vi "Arduino to LabVIEW Communication Module JSON.vi"() -> ()   [LabVIEW 2018]
uses:
  TypeDeclarations/GEVE Ventilator Monitoring Data.ctl
  <vilib>/Instr/_visa.llb/VISA Configure Serial Port (Instr).vi
panel:
  out "GEVE Ventilator Monitoring Data":T1
  out "loop time (ms)":u32
  out "Waveform Chart":u32(graph)
  out "read buffer data byte array":u8[](array[numeric]) format="%02x"
  in  "baud rate (9600)":u32=9600
  out "Communication Timeout?":bool
  in  "VISA resource name":refnum<visa-resource-name>="COM7"
  out "return count read":u32
  out "read buffer":string
  in  "Stop":bool
  out "Iterations":i32
  # "DEBUG AREA"
  # "iterations"
  # "poti"
  # "pressure"
  # "alarm"
  # "EOL"
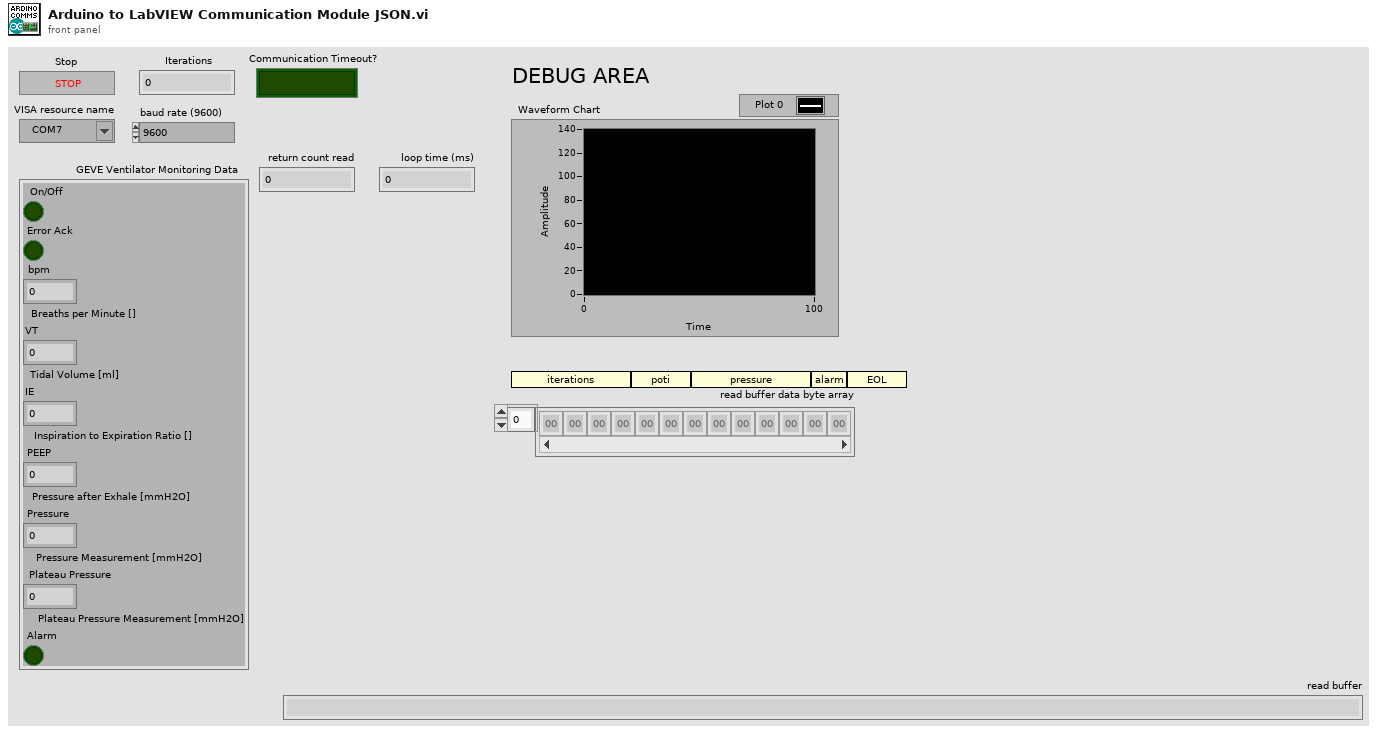
[diagram p1: front panel]
types:
  T1 = typedef "GEVE Ventilator Monitoring Data.ctl" = cluster{"On/Off":bool, "Error Ack":bool, "bpm":dbl, "VT":dbl, "IE":dbl, "PEEP":dbl, "Pressure":dbl, "Plateau Pressure":dbl, "Alarm":bool}
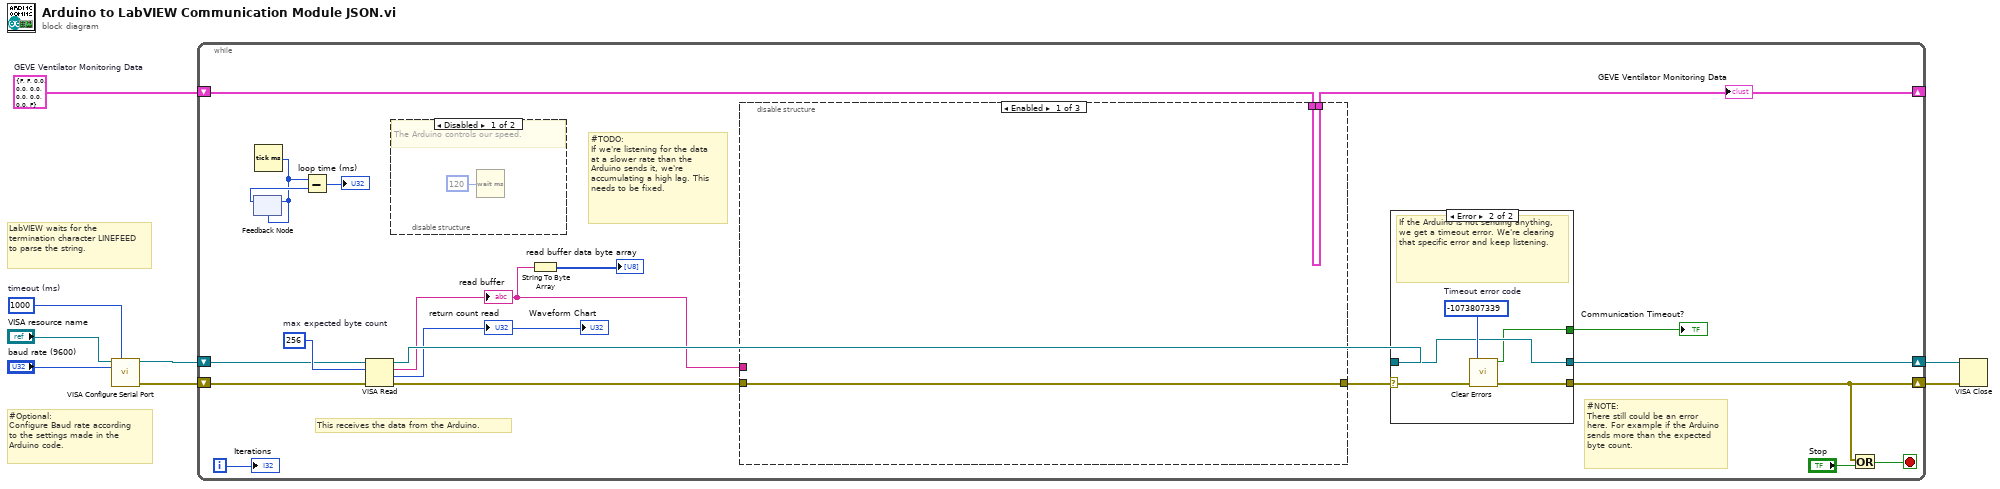
[diagram p0: block diagram]
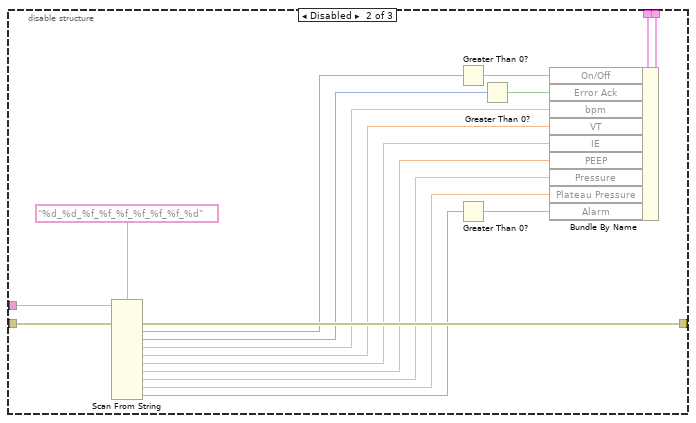
[diagram p2: hidden frame]
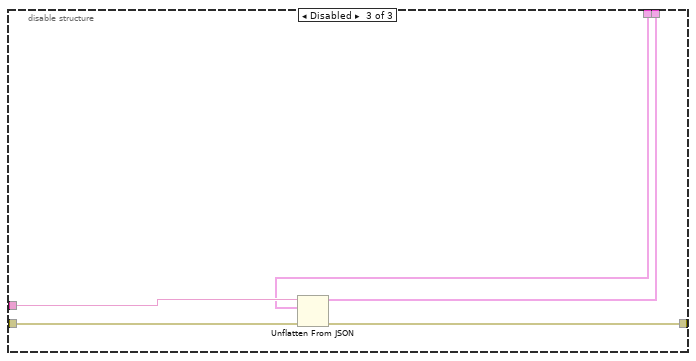
[diagram p3: hidden frame]
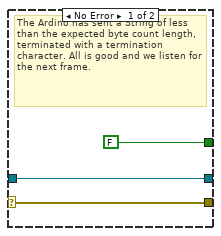
[diagram p5: hidden frame]
diagram:
  w1 = T1 {"On/Off"=FALSE, "Error Ack"=FALSE, "bpm"=0.0, "VT"=0.0, "IE"=0.0, "PEEP"=0.0, "Pressure"=0.0, "Plateau Pressure"=0.0, "Alarm"=FALSE}  # GEVE Ventilator Monitoring Data
  w3 = u32 1000  # timeout (ms)
  # "#Optional:\nConfigure Baud rate according to the settings made in the Arduino code."
  # "LabVIEW waits for the termination character LINEFEED to parse the string."
  n1 = call-poly "VISA Configure Serial Port"("VISA resource name"="VISA resource name", "timeout (10sec)"=w3, "baud rate (9600)"="baud rate (9600)") -> ("VISA resource name out"=w8:refnum<visa-resource-name>, "error out"=w6:errorcluster)  [unwired: 11 in]
  n2 = while {
    shift-right: [w23] -> w7
    shift-left: w8 -> [w12]
    shift-right: [w24] -> w5
    shift-left: w6 -> [w11]
    shift-right: [w9] -> _
    shift-left: w1 -> [w10]
    i -> [w28]
    stop <- w26 stop-if-true
    w25 = u32 256  # max expected byte count
    # "#TODO:\nIf we're listening for the data at a slower rate than the Arduino sends it, we're accumulating a high lag. This needs to be fixed."
    # "This receives the data from the Arduino."
    # "#NOTE:\nThere still could be an error here. For example if the Arduino sends more than the expected byte count."
    n3 = Tick Count (ms)() -> (millisecond timer value=w13:u32)
    n4 = feedback #1(w13) -> (w15:u32)
    n5 = feedback-in #1(w13) -> ()
    n6 = Subtract(x=w13, y=w15) -> (x-y=→"loop time (ms)":u32)
    n7 = VISA Read(VISA resource name=w12, byte count=w25, error in (no error)=w11) -> (VISA resource name out=w22:refnum<visa-resource-name>, read buffer=w17:string, return count=→"return count read" →"Waveform Chart":u32, error out=w16:errorcluster)
    "read buffer" <- w17
    n8 = disable-structure shown="Disabled" {
      frame Disabled {
        # "The Arduino controls our speed."
        n9 = Wait (ms)(milliseconds to wait=u32 120) -> ()  [unwired: 1 out]
      }
      frame Enabled {
      }
    }
    n10 = String To Byte Array(string=w17) -> (unsigned byte array=→"read buffer data byte array":u8[])
    n11 = disable-structure shown="Enabled" {
      disable-tunnel: [w30 w48 w52] -> w20
      disable-tunnel: w17 -> [_ w47 w51]
      disable-tunnel: w16 -> [w30 w46 w53]
      disable-tunnel: w10 -> [w29 w43 w50]
      disable-tunnel: [w29 w42 w49] -> w9
      frame Enabled {
      }
      frame Disabled {
        n12 = Scan From String(format string="%d_%d_%f_%f_%f_%f_%f_%f_%d", input string=w47, error in=w46) -> (error out=w48:errorcluster, output 1=w40:i32, output 2=w39:i32, output 3=w44:dbl, output 4=w31:dbl, output 5=w32:dbl, output 6=w33:dbl, output 7=w34:dbl, output 8=w35:dbl, output 9=w41:i32)  [unwired: 10 in, 2 out]
        n13 = Greater Than 0?(x=w40) -> (x > 0?=w38:bool)
        n14 = Greater Than 0?(x=w41) -> (x > 0?=w36:bool)
        n15 = Greater Than 0?(x=w39) -> (x > 0?=w37:bool)
        n16 = Bundle By Name(cluster=w43, "On/Off"=w38, "Error Ack"=w37, "bpm"=w44, "VT"=w31, "IE"=w32, "PEEP"=w33, "Pressure"=w34, "Plateau Pressure"=w35, "Alarm"=w36) -> (w42:T1)
      }
      frame Disabled {
        n17 = Unflatten From JSON(JSON string=w51, type and defaults=w50, error in (no error)=w53) -> (value=w49:T1, error out=w52:errorcluster)  [unwired: 4 in]
      }
    }
    "GEVE Ventilator Monitoring Data" <- w9
    n18 = case shown="Error" w20 {
      selector: w20 -> [w57 w62]
      tunnel: [w57 w60] -> w24
      tunnel: [w56 w59] -> w23
      tunnel: w22 -> [w56 w59]
      tunnel: [FALSE ("specific error cleared?") w58] -> w21
      frame No Error {
        # "The Ardino has sent a String of less than the expected byte count length, terminated with a termination character. All is good and we listen for the next frame."
      }
      frame Error {
        w61 = -1073807339  # Timeout error code
        # "If the Arduino is not sending anything, we get a timeout error. We're clearing that specific error and keep listening."
        n19 = call <vilib>:"Clear Errors.vi"("error in (no error)"=w62, "specific error code to clear (0: all)"=w61) -> ("error out"=w60:errorcluster, "specific error cleared?"=w58:bool)  [unwired: 4 in]
      }
    }
    "Communication Timeout?" <- w21
    n20 = Or(x=w24, y="Stop") -> (x .or. y?=w26:bool)
    "Iterations" <- w28
  }
  n21 = VISA Close(VISA resource name=w7, error in (no error)=w5) -> ()  [unwired: 1 out]
